vi "Manager Executable Post-Build Action.vi"(5 "Files Generated by Build":path[](array[path]), 6 "Top Level/Always Included VIs":path[](array[path]), 7 "Destination Path":path, 8 "error in (no error)":errorcluster, 9 "Target Name":string, 10 "Build Specification Name":string, 11 "Project Path":path) -> (0 "error out":errorcluster)   [LabVIEW 2021, in "CIF Build Actions.lvlib"]
uses:
  CIF Build Actions.lvlib
  CIFConfigurationFile/typedef/Location Type.ctl
  CIFConfigurationFile/CIF Configuration File Location.vi
  <vilib>/CIF Foundation/CIF Utilities/File/File/Prune to Directory.vi
  <vilib>/Utility/error.llb/Clear Errors.vi
  <vilib>/Utility/libraryn.llb/Check if File or Folder Exists.vi
  <vilib>/regexp/Match Regular Expression.xnode
  <vilib>/CIF Foundation/CIF Utilities/File/File_CIF_U.lvlib
  CIFConfigurationFile/CIF Configuration File.lvlib
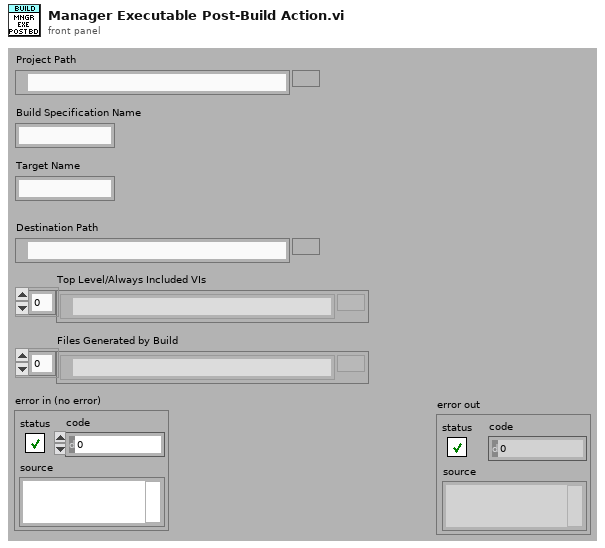
[diagram p1: front panel]
types:
  T1 = typedef "CIF Configuration File.lvlib/Location Type.ctl" = enum16{"Config File", "Manager", "Protos", "Plugins", "UI Plugins", "Logs", "Orchestrations"}
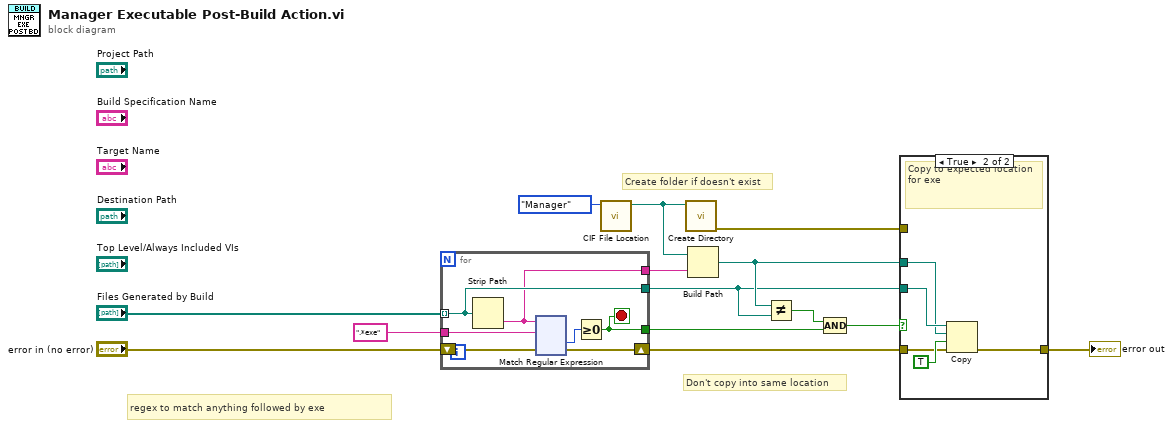
[diagram p0: block diagram]
diagram:
  # "Create folder if doesn't exist"
  # "Don't copy into same location"
  # "regex to match anything followed by exe"
  n1 = for {
    tunnel: "Files Generated by Build" -> [w20] mode=indexing
    tunnel: ".*exe" ("pattern") -> [w21]
    tunnel: [w20] -> w7
    tunnel: [w18] -> w12
    shift-right: [w16] -> w10
    shift-left: "error in (no error)" -> [w17]
    tunnel: [w15] -> w6
    stop <- w15 stop-if-true
    n2 = Strip Path(path=w20) -> (name=w18:string)  [unwired: 1 out]
    n3 = xnode "Match Regular Expression"("input string"=w18, "regular expression"=w21, "error in"=w17) -> ("offset past match"=w19:i32, "error out"=w16:errorcluster)  [unwired: 3 in, 3 out]
    n4 = Greater Or Equal To 0?(x=w19) -> (x >= 0?=w15:bool)
  }
  n5 = call "CIF File Location.vi"("LocationType"=Location_Type."Manager") -> ("Location"=w1:path)  [unwired: 10 in]
  n6 = call <vilib>:"Create Directory.vi"("Path In"=w1) -> ("error out"=w3:errorcluster)  [unwired: 9 in, 1 out]
  n7 = Build Path(base path=w1, name or relative path=w12) -> (appended path=w8:path)
  n8 = Not Equal?(x=w8, y=w7) -> (x != y?=w5:bool)
  n9 = Compound Arithmetic op=AND(w5, w6) -> (w4:bool)
  n10 = case shown="True" w4 {
    tunnel: w7 -> [_ w144]
    tunnel: w8 -> [_ w143]
    tunnel: w10 -> [w139 w141]
    tunnel: [w139 w140] -> w9
    tunnel: w3 -> [_ _]
    frame False {
      # "PPL not found, could provide error"
    }
    frame True {
      # "Copy to expected location for exe"
      n11 = Copy(8:w141, 9:TRUE ("overwrite (F)"), 10:w143, 11:w144) -> (0:w140:errorcluster)  [unwired: 1 in, 2 out]
    }
  }
  "error out" <- w9
